vi "Read xPointingCorrection_arcsec.vi"(8 "error in (no error)":errorcluster, 11 "ADCPointingCorrectionOffsets in":refnum<class "ADCPointingCorrectionOffsets.lvclass">) -> (0 "error out":errorcluster, 2 "xPointingCorrection_arcsec":dbl[unit] min=-0.0048481368110953596 max=0.0048481368110953596, 3 "ADCPointingCorrectionOffsets out":refnum<class "ADCPointingCorrectionOffsets.lvclass">)   [LabVIEW 2022 SP3, in "TCSDataDefinitions.lvlib" / "TCSAtmosphericDispersionCommand.lvlib" / "ADCPointingCorrectionOffsets.lvclass"]
uses:
  ADCPointingCorrectionOffsets.lvclass
  ADCPointingCorrectionOffsets.lvclass/ADCPointingCorrectionOffsets.ctl
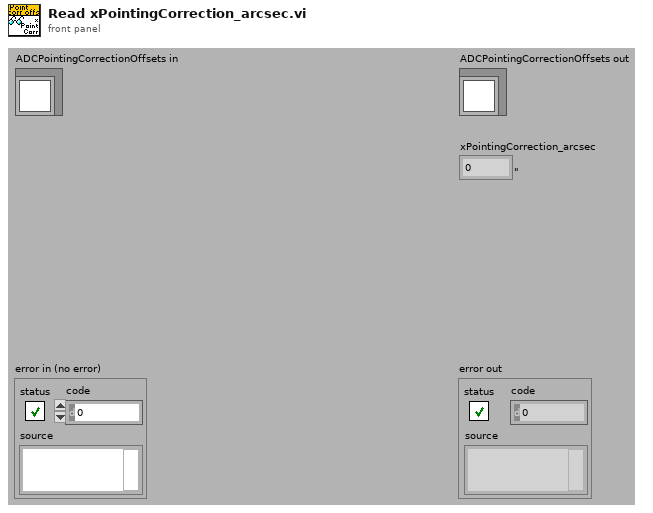
[diagram p1: front panel]
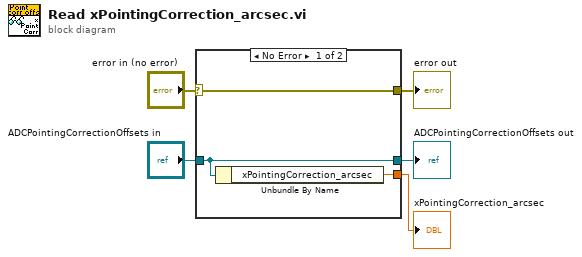
[diagram p0: block diagram]
diagram:
  n1 = case shown="No Error" "error in (no error)" {
    selector: "error in (no error)" -> [w8 w9]
    tunnel: [w8 w9] -> w4
    tunnel: [w7 w10] -> w2
    tunnel: "ADCPointingCorrectionOffsets in" -> [w7 w10]
    tunnel: [w6 _] -> w1
    frame No Error {
      n2 = Unbundle By Name(w7) -> ("xPointingCorrection_arcsec"=w6:dbl[unit])
    }
    frame Error {
    }
  }
  "error out" <- w4
  "ADCPointingCorrectionOffsets out" <- w2
  "xPointingCorrection_arcsec" <- w1
